vi "getInheritanceChain.vi"(8 "error in (no error)":errorcluster, 11 "Tree in":refnum<class "Tree.lvclass">) -> (0 "error out":errorcluster, 2 "Inheritance Chain":string[](array[string]), 3 "Tree out":refnum<class "Tree.lvclass">)   [LabVIEW 2009, in "Tree.lvclass"]
doc: "Returns the inheritance chain."
uses:
  Tree.lvclass
  Structure/Structure.lvclass
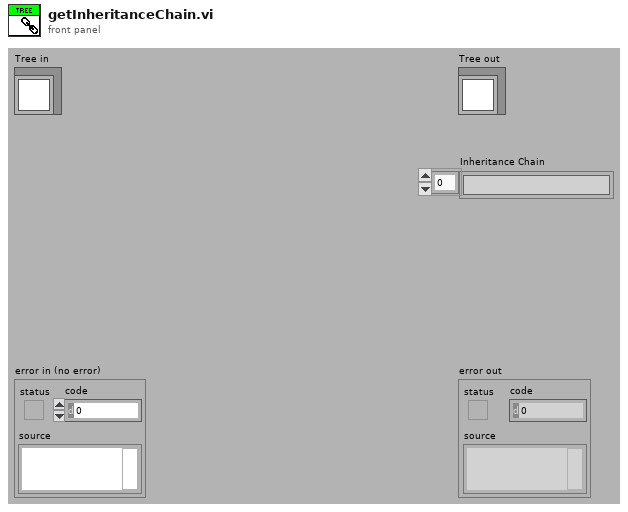
[diagram p1: front panel]
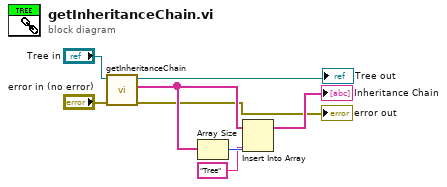
[diagram p0: block diagram]
diagram:
  n1 = call-parent "getInheritanceChain.vi"("error in (no error)"="error in (no error)", "Structure in"="Tree in") -> ("error out"=→"error out":errorcluster, "Inheritance Chain"=w4:string[], "Structure out"=→"Tree out":refnum<class "Tree.lvclass">)  [unwired: 7 in]
  n2 = Array Size(array=w4) -> (size(s)=w6:i32)
  n3 = Insert Into Array(array=w4, index=w6, new element="Tree") -> (→"Inheritance Chain":string[])
